vi "Multiply Float SCTL 40 MHz Latency 0 Pipeline 0.vi"(1 "y":sgl, 2 "x":sgl) -> (0 "x*y":sgl)   [LabVIEW 2014]
uses:
  <vilib>/rvi/IPIntegrationNode/IPINode_Typedef/niFpgaIPINodeSupportedFamilies.ctl
  <vilib>/rvi/IPIntegrationNode/IPINode_Utilities/niFpgaIPINodeSimCore.vi
  <vilib>/rvi/XilinxIP/XIPIN_XNode/niFpgaXIPIN.xnode
  Coregen KINTEX7/Multiply SCTL L0/xsim.dir/Multiply_SCTL_L0_91721A02967D4925A2B5FA29BCD18B30/xsimk_91721A02967D4925A2B5FA29BCD18B30.dll
  <vilib>/rvi/IPIntegrationNode/IPINode_Xnode/niFpgaIPINode.xnode
  Coregen SPARTAN6/Multiply SCTL L0/Multiply_SCTL_L0_C3ADE5BE76064AA39E7EE6565DE88692.dll
  Coregen Zynq/Multiply SCTL L0/xsim.dir/Multiply_SCTL_L0_184E08AD97044BA3AD7104FB20BDBA66/xsimk_184E08AD97044BA3AD7104FB20BDBA66.dll
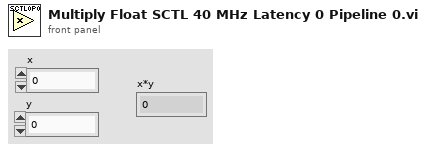
[diagram p1: front panel]
types:
  T1 = typedef "niFpgaIPINodeSupportedFamilies.ctl" = cluster{"unlimited?":bool, "supported targets":string[]}
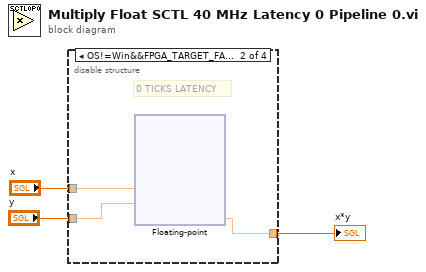
[diagram p0: block diagram]
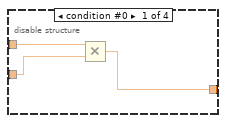
[diagram p2: hidden frame]
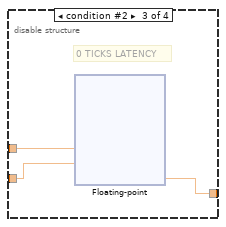
[diagram p3: hidden frame]
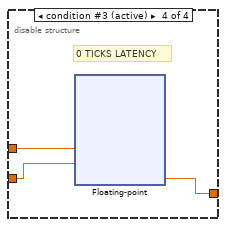
[diagram p4: hidden frame]
diagram:
  n1 = disable-structure shown="OS!=Win&&FPGA_TARGET_FAMILY==SPARTAN6" {
    disable-tunnel: "x" -> [w6 w9 w66 w129]
    disable-tunnel: "y" -> [w5 w8 w64 w127]
    disable-tunnel: [w4 w7 w65 w128] -> w1
    frame condition #0 {
      n2 = Multiply(x=w6, y=w5) -> (x*y=w4:sgl)
    }
    frame condition #1 {
      # "0 TICKS LATENCY"
      n3 = xnode ("Floating-point")("a"=w9, "b"=w8) -> ("result"=w7:sgl)
    }
    frame condition #2 {
      # "0 TICKS LATENCY"
      n4 = xnode ("Floating-point")("s_axis_a_tdata"=w66, "s_axis_b_tdata"=w64) -> ("m_axis_result_tdata"=w65:sgl)  [unwired: 2 in, 1 out]
    }
    frame condition #3 (active) {
      # "0 TICKS LATENCY"
      n5 = xnode ("Floating-point")("s_axis_a_tdata"=w129, "s_axis_b_tdata"=w127) -> ("m_axis_result_tdata"=w128:sgl)  [unwired: 2 in, 1 out]
    }
  }
  "x*y" <- w1
